vi "Get Next.vi"(7 "Unique ID":string, 8 "error in (no error)":errorcluster, 11 "Test Executive Ref":refnum<data-value>) -> (0 "error out":errorcluster, 1 "Test":refnum<class "Executioner.lvclass">, 2 "Active Test Executive Ref out":refnum<data-value>, 3 "Test Executive Ref out":refnum<data-value>, 4 "Found":bool, 5 "Unique ID out":string, 6 "Complete":bool)   [LabVIEW 2019, in "Test Executive.lvlib" / "TestExecutive Ref.lvclass"]
uses:
  <vilib>/gpm_packages/@cs/test-executive/Source/Test Executive/TestExecutive Ref/TestExecutive Ref.lvclass
  <vilib>/gpm_packages/@cs/test-executive/Source/Test Executive/ITestExecutive/ITest Executive.lvclass
  <vilib>/gpm_packages/@cs/test-executive/Source/Test Executive/Executioner/Executioner.lvclass
panel:
  # "Need some documentation on\nwhat this is for (it's for subroutines)"
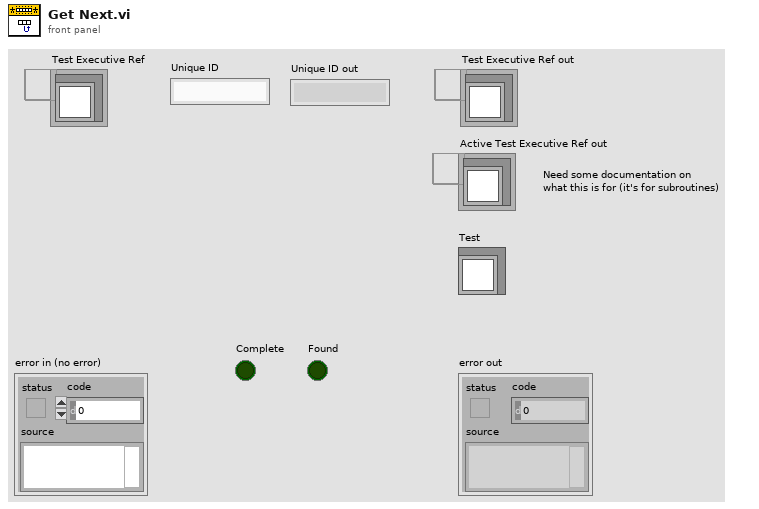
[diagram p1: front panel]
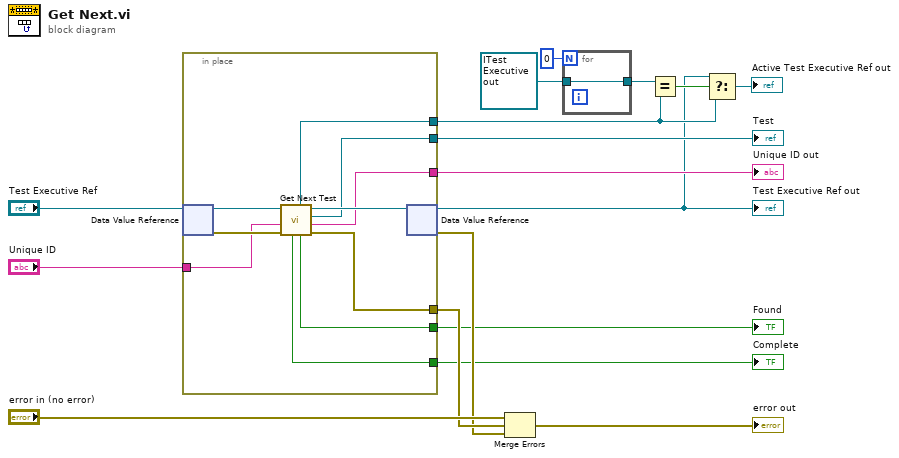
[diagram p0: block diagram]
diagram:
  n1 = in-place {
    in-place-border: "Unique ID" -> [w23]
    in-place-border: [w22] -> w15
    in-place-border: [w26] -> w13
    in-place-border: [w21] -> w10
    in-place-border: [w20] -> w9
    in-place-border: [w19] -> w8
    in-place-border: [w18] -> w3
    n2 = in-place-dvr #1("Test Executive Ref") -> (w25:refnum<class "ITest Executive.lvclass">, w27:errorcluster)
    n3 = call-dynamic "Get Next Test.vi"("error in (no error)"=w27, "Active Unique ID"=w23, "ITest Executive in"=w25) -> ("error out"=w26:errorcluster, "Active Unique ID out"=w22:string, "Test"=w21:refnum<class "Executioner.lvclass">, "ITest Executive out"=w24:refnum<class "ITest Executive.lvclass">, "Found"=w20:bool, "Test Executive Ref out"=w18:refnum<data-value>, "Complete"=w19:bool)  [unwired: 2 in]
    n4 = in-place-dvr #1(w24) -> (w2:refnum<data-value>, w12:errorcluster)
  }
  "Test Executive Ref out" <- w2
  "Unique ID out" <- w15
  "Test" <- w10
  "Found" <- w9
  "Complete" <- w8
  n5 = Merge Errors("error in (no error)", w13, w12) -> (→"error out":errorcluster)
  n6 = for {
    N: 0 -> [_]
    tunnel: refnum<data-value> refnum ("Test Executive Ref out") -> [w28]
    tunnel: [w28] -> w5
  }
  n7 = Equal?(x=w5, y=w3) -> (x = y?=w4:bool)
  n8 = Select(t=w2, s=w4, f=w3) -> (s? t:f=→"Active Test Executive Ref out":refnum<data-value>)
